vi "Position Main Tab.vi"(8 "error in (no error)":errorcluster, 10 "Splitter Refnum":refnum<vi>, 11 "TabCtl Refnum":refnum<vi>) -> (0 "error out":errorcluster)   [LabVIEW 2014]
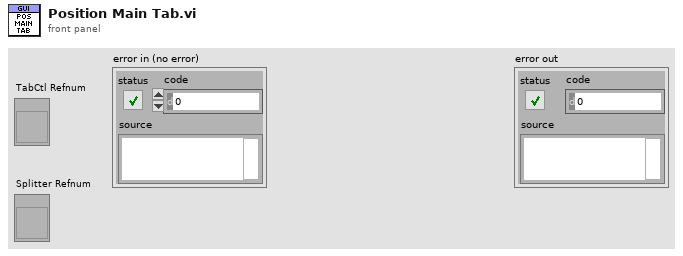
[diagram p1: front panel]
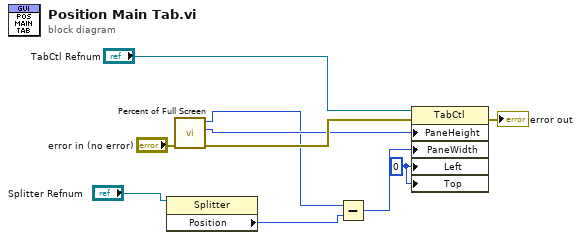
[diagram p0: block diagram]
diagram:
  w1 = 0 ("Position:Left")
  n1 = property class="Splitter"(reference="Splitter Refnum") -> ("Position"=w4:i32)  [unwired: 1 in, 2 out]
  n2 = call "Percent of Full Screen.vi"("error in (no error)"="error in (no error)") -> ("error out"=w9:errorcluster, "Bottom"=w8:i16, "Right"=w5:i16)  [unwired: 8 in]
  n3 = Subtract(x=w5, y=w4) -> (x-y=w3:i32)
  n4 = property class="TabCtl"(reference="TabCtl Refnum", error in=w9, "PaneHeight"=w8, "PaneWidth"=w3, "Left"=w1, "Top"=w1) -> (error out=→"error out":errorcluster)  [unwired: 1 out]
